vi "Sub_Preprocessing_FEA_Populate_Matrix.vi"(10 "No. of Nodes":i32, 11 "Element Matrix":dbl[][](array[numeric])) -> (3 "Matrix w/o BC":dbl[][](array[numeric]))   [LabVIEW 2021]
panel:
  in  "Modeling Parameters":T1
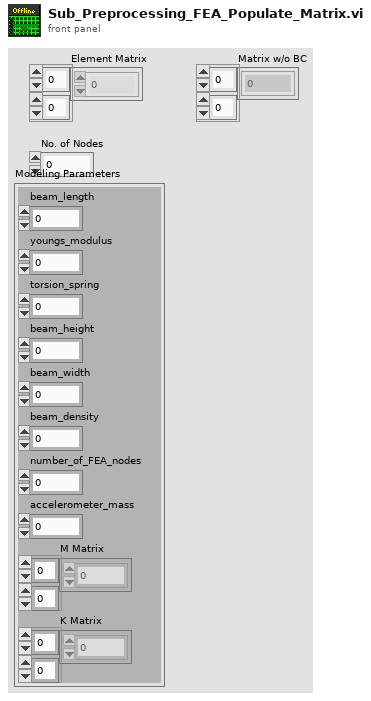
[diagram p1: front panel]
types:
  T1 = cluster{"beam_length":dbl, "youngs_modulus":dbl, "torsion_spring":dbl, "beam_height":dbl, "beam_width":dbl, "beam_density":dbl, "number_of_FEA_nodes":i32, "accelerometer_mass":dbl, "M Matrix":dbl[][], "K Matrix":dbl[][]}
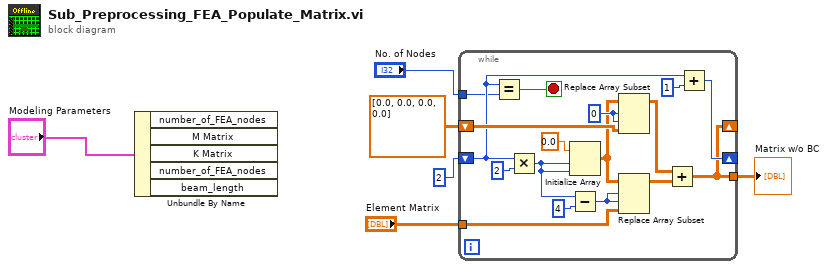
[diagram p0: block diagram]
diagram:
  n1 = Unbundle By Name("Modeling Parameters") -> ()  [unwired: 5 out]
  n2 = while {
    shift-right: [w9] -> _
    shift-left: dbl[][] [[0.0, 0.0], [0.0, 0.0]] -> [w20]
    shift-right: [w16] -> _
    shift-left: 2 -> [w13]
    tunnel: "No. of Nodes" -> [w12]
    tunnel: "Element Matrix" -> [w10]
    tunnel: [w9] -> w5
    stop <- w11 stop-if-true
    w19 = 0 ("index")
    n3 = Equal?(x=w13, y=w12) -> (x = y?=w11:bool)
    n4 = Multiply(x=w13, y=2) -> (x*y=w8:i32)
    n5 = Initialize Array(0.0 ("element"), w8, w8) -> (w7:dbl[][])
    n6 = Subtract(x=w8, y=4) -> (x-y=w18:i32)
    n7 = Replace Array Subset(array=w7, new element=w20, index (row)=w19, index (col)=w19) -> (w15:dbl[][])
    n8 = Replace Array Subset(array=w7, new element=w10, index (row)=w18, index (col)=w18) -> (w14:dbl[][])
    n9 = Add(x=w15, y=w14) -> (x+y=w9:dbl[][])
    n10 = Add(x=w13, y=1) -> (x+y=w16:i32)
  }
  "Matrix w/o BC" <- w5
